vi "ParseCaps.vi"(8 "error in (no error)":errorcluster, 11 "caps file text":string) -> (0 "error out":errorcluster, 2 "Caps":T1, 3 "json caps":string)   [LabVIEW 2017, in "Paser.lvlib"]
doc: "<B>This VI is used for parsing JSON text and binding Registers with Properties.</B>"
uses:
  API/Parser/Paser.lvlib
  Ctrl/Caps.ctl
  Ctrl/Property.ctl
  Ctrl/PhysicalChannel.ctl
  Ctrl/Register.ctl
  Ctrl/Bitfield.ctl
  Ctrl/Scale.ctl
  Ctrl/ScaleType.ctl
  Ctrl/Enum.ctl
  Ctrl/EnumValue.ctl
  8a91daa8-18c1-4d98-a5cc-92a44b2a1c41.vi
  <vilib>/JDP Science/JSONtext/Find Item.vi
  <vilib>/JDP Science/JSONtext/String Subset.vi
  <vilib>/JDP Science/JSONtext/Parsing/Parse Full Path or Item Name.vi
  <vilib>/JDP Science/JSONtext/Offset/Find Item Locations by Path.vi
  <vilib>/JDP Science/JSONtext/JSON text to Variant.vi
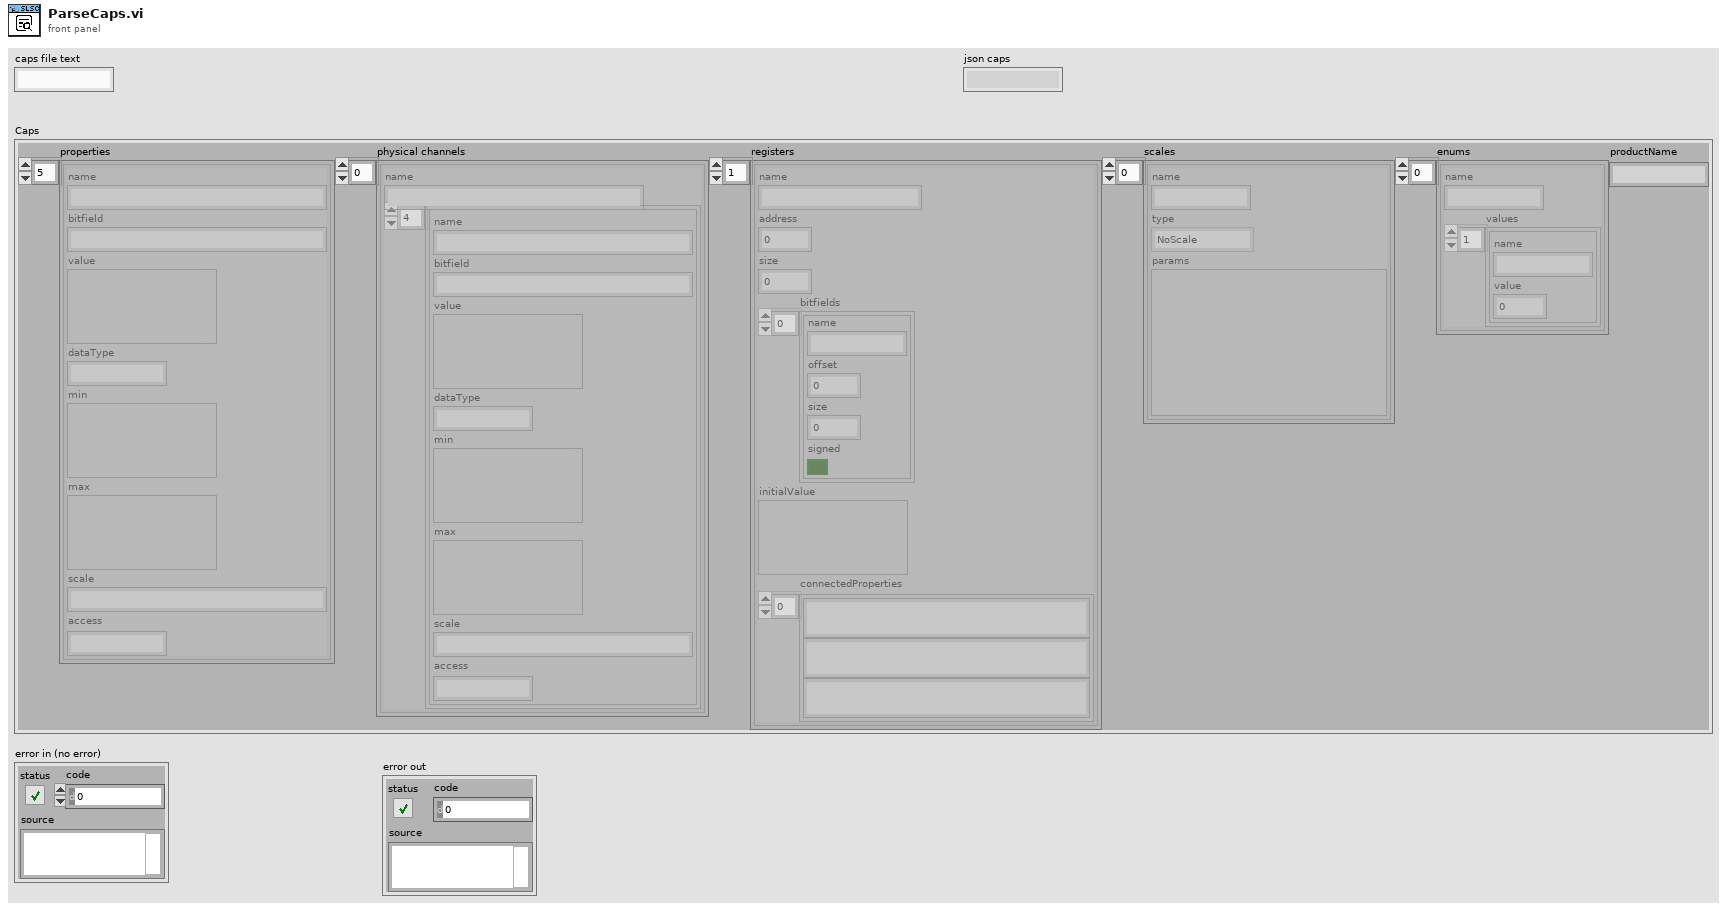
[diagram p1: front panel]
types:
  T1 = typedef "Caps.ctl" = cluster{"properties":T2[], "physical channels":T3[], "registers":T4[], "scales":T6[], "enums":T8[], "productName":string}
  T2 = typedef "Property.ctl" = cluster{"name":string, "bitfield":string, "value":variant, "dataType":string, "min":variant, "max":variant, "scale":string, "access":string}
  T3 = typedef "PhysicalChannel.ctl" = cluster{"name":string, "properties":T2[]}
  T4 = typedef "Register.ctl" = cluster{"name":string, "address":i32, "size":i32, "bitfields":T5[], "initialValue":variant, "connectedProperties":string[]}
  T5 = typedef "Bitfield.ctl" = cluster{"name":string, "offset":i32, "size":i32, "signed":bool}
  T6 = typedef "Scale.ctl" = cluster{"name":string, "type":T7, "params":variant}
  T7 = typedef "ScaleType.ctl" = enum16{"NoScale", "Table", "Polynomial", "Linear"}
  T8 = typedef "Enum.ctl" = cluster{"name":string, "values":T9[]}
  T9 = typedef "EnumValue.ctl" = cluster{"name":string, "value":i32}
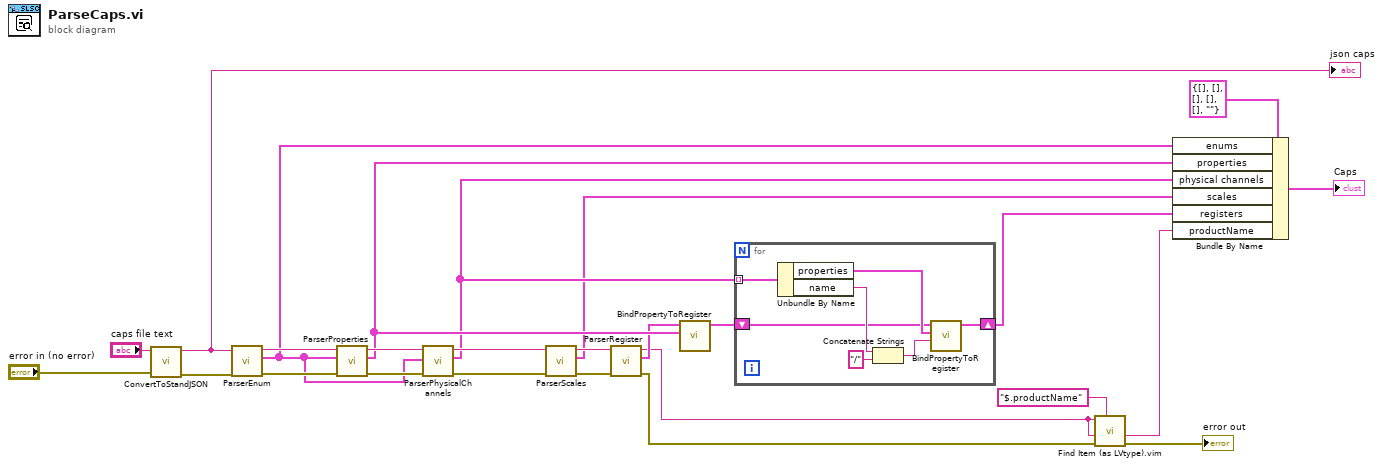
[diagram p0: block diagram]
diagram:
  n1 = call "ConvertToStandJSON.vi"("error in (no error)"="error in (no error)", "caps"="caps file text") -> ("error out"=w10:errorcluster, "json caps"=w12:string)  [unwired: 8 in]
  "json caps" <- w12
  n2 = call "ParserEnum.vi"("error in (no error)"=w10, "JSON item"=w12) -> ("error out"=w9:errorcluster, "enums"=w7:T8[], "JSON item"=w11:string)  [unwired: 7 in]
  n3 = call "ParserProperties.vi"("error in (no error)"=w9, "enums"=w7, "JSON item"=w11) -> ("error out"=w26:errorcluster, "properties"=w19:T2[], "JSON item"=w25:string)  [unwired: 4 in]
  n4 = call "ParserPhysicalChannels.vi"("error in (no error)"=w26, "enums"=w7, "JSON item"=w25) -> ("error out"=w23:errorcluster, "physical channels"=w18:T3[], "JSON item"=w24:string)  [unwired: 6 in]
  n5 = call "ParserScales.vi"("error in (no error)"=w23, "JSON item"=w24) -> ("error out"=w21:errorcluster, "scales"=w1:T6[], "JSON item"=w22:string)  [unwired: 7 in]
  n6 = call "ParserRegister.vi"("error in (no error)"=w21, "JSON item"=w22) -> ("error out"=w3:errorcluster, "registers"=w17:T4[], "JSON item"=w8:string)  [unwired: 7 in]
  n7 = call "BindPropertyToRegister.vi"("properties"=w19, "registers"=w17) -> ("registers"=w20:T4[])  [unwired: 9 in]
  n8 = for {
    tunnel: w18 -> [w33] mode=indexing
    shift-right: [w29] -> w2
    shift-left: w20 -> [w27]
    n9 = Unbundle By Name(w33) -> ("properties"=w28:T2[], "name"=w30:string)
    n10 = Concatenate Strings(w30, "/" ("string")) -> (w32:string)
    n11 = call "BindPropertyToRegister.vi"("context"=w32, "properties"=w28, "registers"=w27) -> ("registers"=w29:T4[])  [unwired: 8 in]
  }
  n12 = call "Find Item (as LVtype).vim"("$Path or Item Name"="$.productName" ("JSON"), "error in (no error)"=w3, "Data Type and Default Value"=w8, "JSON"=w8) -> ("error out"=→"error out":errorcluster, "Data"=w13:string)  [unwired: 4 in, 2 out]
  n13 = Bundle By Name(cluster=T1 {"properties"=[], "physical channels"=[], "registers"=[], "scales"=[], "enums"=[], "productName"=""} ("Caps"), "enums"=w7, "properties"=w19, "physical channels"=w18, "scales"=w1, "registers"=w2, "productName"=w13) -> (→"Caps":T1)
